vi "Configure PLC Remote.vi"(8 "error IO":errorcluster, 10 "PLC Remote":bool, 11 "VISA resource name":refnum<visa-resource-name>) -> (0 "error Out":errorcluster, 3 "VISA resource Out":refnum<visa-resource-name>)   [LabVIEW 2020, in "eec EST 300.lvlib"]
doc: "Specify where the trigger source to perform test.\n\nValid Range: \nTrue: Test could only be Triggered from Remote IO.\nFalse: Test could only be Triggered from \"TEST\" button on panel."
uses:
  <instrlib>/eec EST 300/eec EST 300.lvlib
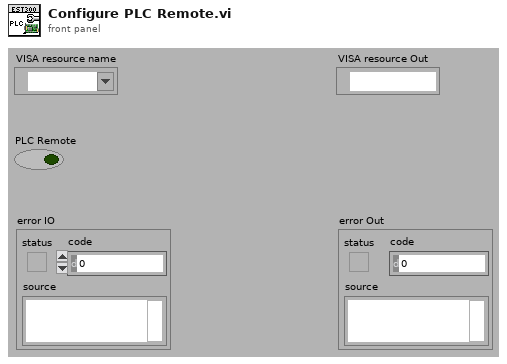
[diagram p1: front panel]
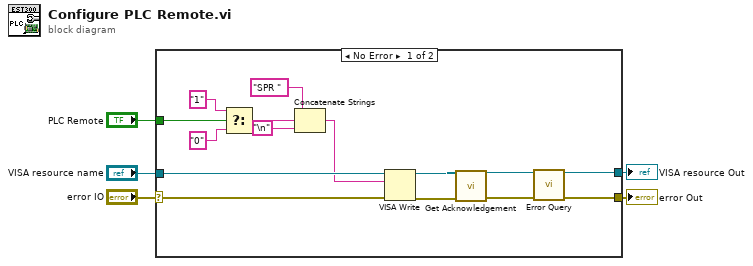
[diagram p0: block diagram]
diagram:
  n1 = case shown="No Error" "error IO" {
    selector: "error IO" -> [w20 w22]
    tunnel: [w17 w22] -> w2
    tunnel: [w18 w21] -> w3
    tunnel: "VISA resource name" -> [w19 w21]
    tunnel: "PLC Remote" -> [w9 _]
    frame No Error {
      n2 = Select(t="1" ("string"), s=w9, f="0" ("string")) -> (s? t:f=w8:string)
      n3 = Concatenate Strings("SPR " ("Command to Send (empty)"), w8, "\n") -> (w14:string)
      n4 = VISA Write(VISA resource name=w19, write buffer=w14, error in (no error)=w20) -> (VISA resource name out=w7:refnum<visa-resource-name>, error out=w6:errorcluster)  [unwired: 1 out]
      n5 = call <instrlib>:"Get Acknowledgement.vi"("VISA resource name"=w7, "error in (no error)"=w6) -> ("VISA resource name out"=w13:refnum<visa-resource-name>, "error out"=w12:errorcluster)  [unwired: 12 in]
      n6 = call <instrlib>:"Error Query.vi"("VISA resource name"=w13, "error in (no error)"=w12) -> ("VISA resource name out"=w18:refnum<visa-resource-name>, "error out"=w17:errorcluster)  [unwired: 10 in, 2 out]
    }
    frame Error {
    }
  }
  "VISA resource Out" <- w3
  "error Out" <- w2
